vi "Is Anchor ID Unique.vi"(2 "Anchor.lvclass":refnum<class "Anchor.lvclass">, 3 "Input AnchorArray":refnum<class "Anchor.lvclass">[](array[class])) -> (17 "Is unique?":bool)   [LabVIEW 2014]
doc: "This VI checks if given Anchor has an unique ID compared to the input Anchor object array."
uses:
  Anchor.lvclass
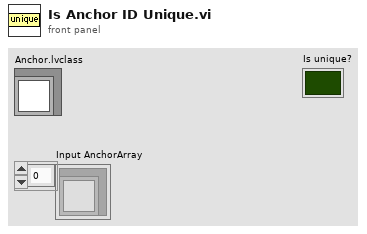
[diagram p1: front panel]
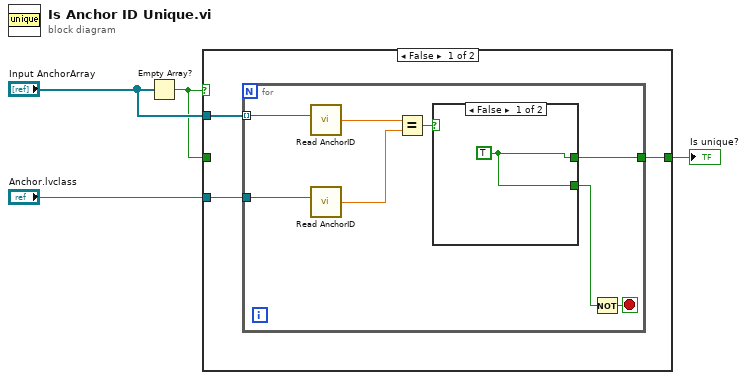
[diagram p0: block diagram]
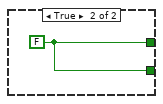
[diagram p2: hidden frame]
diagram:
  n1 = Empty Array?(array="Input AnchorArray") -> (empty?=w2:bool)
  n2 = case shown="False" w2 {
    tunnel: "Anchor.lvclass" -> [w6 _]
    tunnel: "Input AnchorArray" -> [w7 _]
    tunnel: w2 -> [_ w18]
    tunnel: [w5 w18] -> w1
    frame False {
      n3 = for {
        tunnel: w7 -> [w15] mode=indexing
        tunnel: w6 -> [w14]
        tunnel: [w8] -> w5
        stop <- w9 stop-if-true
        n4 = call-dynamic "Read AnchorID.vi"("Anchor in"=w15) -> ("AnchorID"=w13:dbl)  [unwired: 1 in, 2 out]
        n5 = call-dynamic "Read AnchorID.vi"("Anchor in"=w14) -> ("AnchorID"=w12:dbl)  [unwired: 1 in, 2 out]
        n6 = Equal?(x=w13, y=w12) -> (x = y?=w11:bool)
        n7 = case shown="False" w11 {
          tunnel: [w16 w17] -> w10
          tunnel: [w16 w17] -> w8
          frame False {
            w16 = TRUE
          }
          frame True {
            w17 = FALSE
          }
        }
        n8 = Not(x=w10) -> (.not. x?=w9:bool)
      }
    }
    frame True {
      # "if array is empty, Anchor is unique by default"
    }
  }
  "Is unique?" <- w1
